vi "Final_Project_Arduino_Reader.vi"() -> ()   [LabVIEW 2017]
uses:
  <vilib>/Instr/_visa.llb/VISA Configure Serial Port (Instr).vi
panel:
  in  "Minutes Between Samples":i32
  in  "Input Array Byte Count":u32
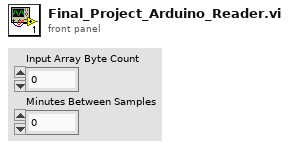
[diagram p1: front panel]
types:
  T1 = enum16{"open", "replace", "create", "open or create", "replace or create", "replace or create with confirmation"}
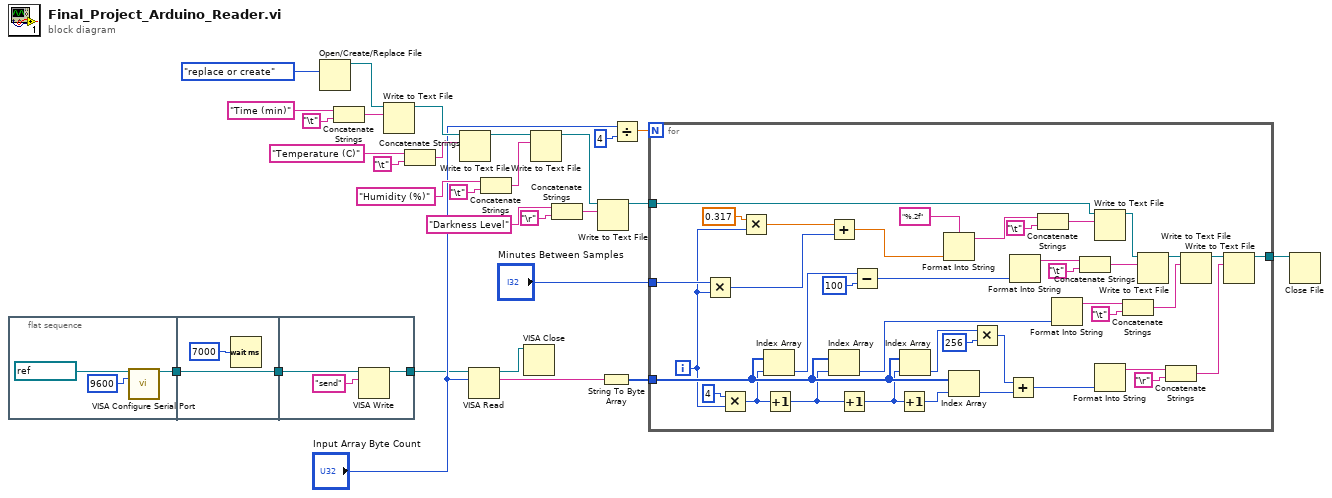
[diagram p0: block diagram]
diagram:
  n1 = flat-sequence {
    tunnel: [w30] -> w2
    tunnel: w2 -> [w34]
    tunnel: [w34] -> w1
    tunnel: w1 -> [w37]
    tunnel: [w36] -> w3
    frame #0 {
      n2 = call-poly "VISA Configure Serial Port"("VISA resource name"=refnum<visa-resource-name> "COM9", "baud rate (9600)"=u32 9600) -> ("VISA resource name out"=w30:refnum<visa-resource-name>)  [unwired: 12 in, 1 out]
    }
    frame #1 {
      n3 = Wait (ms)(milliseconds to wait=7000) -> ()  [unwired: 1 out]
    }
    frame #2 {
      n4 = VISA Write(VISA resource name=w37, write buffer="send") -> (VISA resource name out=w36:refnum<visa-resource-name>)  [unwired: 1 in, 2 out]
    }
  }
  n5 = Open/Create/Replace File(operation (0:open)=T1."replace or create") -> (refnum out=w28:refnum<file>)  [unwired: 5 in, 2 out]
  n6 = Concatenate Strings("Time (min)", "\t") -> (w23:string)
  n7 = Write to Text File(file (use dialog)=w28, text=w23) -> (refnum out=w27:refnum<file>)  [unwired: 2 in, 2 out]
  n8 = Concatenate Strings("Temperature (C)", "\t") -> (w20:string)
  n9 = Write to Text File(file (use dialog)=w27, text=w20) -> (refnum out=w26:refnum<file>)  [unwired: 2 in, 2 out]
  n10 = VISA Read(VISA resource name=w3, byte count="Input Array Byte Count") -> (VISA resource name out=w4:refnum<visa-resource-name>, read buffer=w12:string)  [unwired: 1 in, 2 out]
  n11 = Concatenate Strings("Humidity (%)", "\t") -> (w17:string)
  n12 = VISA Close(VISA resource name=w4) -> ()  [unwired: 1 in, 1 out]
  n13 = Write to Text File(file (use dialog)=w26, text=w17) -> (refnum out=w13:refnum<file>)  [unwired: 2 in, 2 out]
  n14 = Concatenate Strings("Darkness Level", "\r") -> (w14:string)
  n15 = Write to Text File(file (use dialog)=w13, text=w14) -> (refnum out=w7:refnum<file>)  [unwired: 2 in, 2 out]
  n16 = String To Byte Array(string=w12) -> (unsigned byte array=w8:u8[])
  n17 = Divide(x="Input Array Byte Count", y=u32 4) -> (x/y=w9:dbl)
  n18 = for {
    N: w9 -> [_]
    tunnel: w8 -> [w76]
    tunnel: w7 -> [w63]
    tunnel: "Minutes Between Samples" -> [w44]
    tunnel: [w46] -> w5
    i -> [w42]
    n19 = Multiply(x=w44, y=w42) -> (x*y=w43:i32)
    n20 = Multiply(x=4, y=w42) -> (x*y=w74:i32)
    n21 = Multiply(x=0.317, y=w42) -> (x*y=w40:dbl)
    n22 = Index Array(array=w76, index=w74) -> (element=w71:u8)
    n23 = Increment(x=w74) -> (x+1=w73:i32)
    n24 = Add(x=w40, y=w43) -> (x+y=w39:dbl)
    n25 = Index Array(array=w76, index=w73) -> (element=w55:u8)
    n26 = Increment(x=w73) -> (x+1=w72:i32)
    n27 = Subtract(x=w71, y=100) -> (x-y=w69:i32)
    n28 = Increment(x=w72) -> (x+1=w59:i32)
    n29 = Index Array(array=w76, index=w72) -> (element=w53:u8)
    n30 = Format Into String(format string="%.2f", w39) -> (resulting string=w66:string)  [unwired: 2 in, 1 out]
    n31 = Index Array(array=w76, index=w59) -> (element=w52:u8)
    n32 = Multiply(x=w53, y=256) -> (x*y=w51:i32)
    n33 = Add(x=w51, y=w52) -> (x+y=w49:i32)
    n34 = Format Into String(w69) -> (resulting string=w68:string)  [unwired: 3 in, 1 out]
    n35 = Concatenate Strings(w66, "\t") -> (w64:string)
    n36 = Format Into String(w55) -> (resulting string=w58:string)  [unwired: 3 in, 1 out]
    n37 = Concatenate Strings(w68, "\t") -> (w60:string)
    n38 = Write to Text File(file (use dialog)=w63, text=w64) -> (refnum out=w62:refnum<file>)  [unwired: 2 in, 2 out]
    n39 = Format Into String(w49) -> (resulting string=w50:string)  [unwired: 3 in, 1 out]
    n40 = Concatenate Strings(w58, "\t") -> (w56:string)
    n41 = Write to Text File(file (use dialog)=w62, text=w60) -> (refnum out=w61:refnum<file>)  [unwired: 2 in, 2 out]
    n42 = Concatenate Strings(w50, "\r") -> (w48:string)
    n43 = Write to Text File(file (use dialog)=w61, text=w56) -> (refnum out=w47:refnum<file>)  [unwired: 2 in, 2 out]
    n44 = Write to Text File(file (use dialog)=w47, text=w48) -> (refnum out=w46:refnum<file>)  [unwired: 2 in, 2 out]
  }
  n45 = Close File(refnum=w5) -> ()  [unwired: 1 in, 2 out]
